vi "Read.vi"(8 "error in (no error)":errorcluster, 10 "byte count":u32, 11 "PowerSupply_IT6333A in":refnum<class "PowerSupply_IT6333A.lvclass">) -> (0 "error out":errorcluster, 2 "read buffer":string, 3 "PowerSupply_IT6333A out":refnum<class "PowerSupply_IT6333A.lvclass">)   [LabVIEW 2013, in "PowerSupply_IT6333A.lvclass"]
uses:
  PowerSupply_IT6333A.lvclass
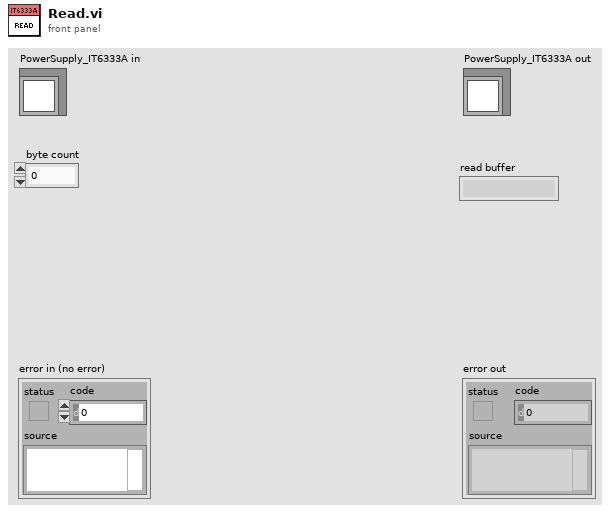
[diagram p1: front panel]
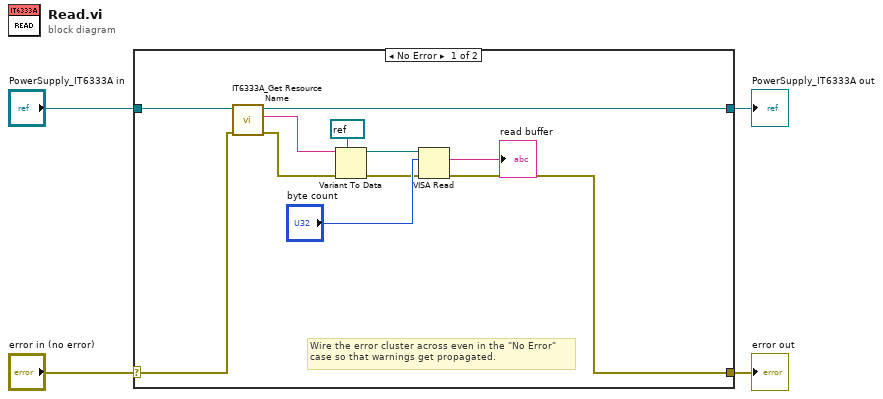
[diagram p0: block diagram]
diagram:
  n1 = case shown="No Error" "error in (no error)" {
    selector: "error in (no error)" -> [w13 w17]
    tunnel: [w12 w17] -> w3
    tunnel: [w14 w16] -> w1
    tunnel: "PowerSupply_IT6333A in" -> [w15 w16]
    frame No Error {
      # "Wire the error cluster across even in the \"No Error\"\ncase so that warnings get propagated."
      n2 = call-dynamic "IT6333A_Get Resource Name.vi"("error in (no error)"=w13, "PowerSupply_IT6333A in"=w15) -> ("error out"=w6:errorcluster, "Resource Name"=w9:string, "PowerSupply_IT6333A out"=w14:refnum<class "PowerSupply_IT6333A.lvclass">)  [unwired: 7 in]
      n3 = Variant To Data(error in=w6, type=refnum<visa-resource-name> refnum ("VISA resource name"), Variant=w9) -> (data=w7:refnum<visa-resource-name>, error out=w5:errorcluster)
      n4 = VISA Read(VISA resource name=w7, byte count="byte count", error in (no error)=w5) -> (read buffer=→"read buffer":string, error out=w12:errorcluster)  [unwired: 2 out]
    }
    frame Error {
    }
  }
  "error out" <- w3
  "PowerSupply_IT6333A out" <- w1
